vi "HTTP-Close.vi"(8 "error in (no error)":errorcluster, 11 "ByteGSWebAPI-V0 in":refnum<class "ByteGSWebAPI-V0.lvclass">) -> (0 "error out":errorcluster, 3 "ByteGSWebAPI-V0 out":refnum<class "ByteGSWebAPI-V0.lvclass">)   [LabVIEW 2019, in "ByteGSWebAPI.lvlib" / "ByteGSWebAPI-V0.lvclass"]
doc: "Ciude la connessione con il server"
uses:
  ByteGSWebAPI-V0.lvclass
  <vilib>/httpClient/ClientHandle.ctl
  ByteGSWebAPI-V0.lvclass/ByteGSWebAPI-V0.ctl
  <vilib>/httpClient/LabVIEWHTTPClient.lvlib
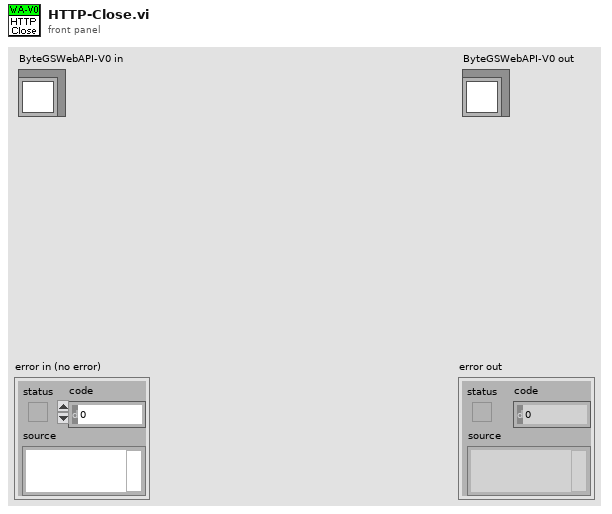
[diagram p1: front panel]
types:
  T1 = typedef "LabVIEWHTTPClient.lvlib/ClientHandle.ctl" = refnum<k1>
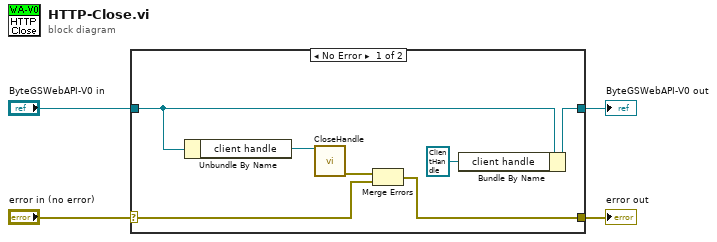
[diagram p0: block diagram]
diagram:
  n1 = case shown="No Error" "error in (no error)" {
    selector: "error in (no error)" -> [w5 w13]
    tunnel: [w6 w13] -> w3
    tunnel: [w9 w12] -> w1
    tunnel: "ByteGSWebAPI-V0 in" -> [w11 w12]
    frame No Error {
      n2 = Unbundle By Name(w11) -> ("client handle"=w10:T1)
      n3 = call <vilib>:"CloseHandle.vi"("client handle"=w10) -> ("error out"=w7:errorcluster)  [unwired: 14 in]
      n4 = Merge Errors(w7, w5) -> (w6:errorcluster)
      n5 = Bundle By Name(cluster=w11, "client handle"=T1 refnum) -> (w9:refnum<class "ByteGSWebAPI-V0.lvclass">)
    }
    frame Error {
    }
  }
  "error out" <- w3
  "ByteGSWebAPI-V0 out" <- w1
